vi "Update Progress bar.vi"(10 "Progress Ref":refnum<vi>, 11 "Measurements In":refnum<class "Measurement.lvclass">) -> (3 "Measurements Out":refnum<class "Measurement.lvclass">)   [LabVIEW 2020, in "Measurement.lvclass"]
uses:
  Measurement.lvclass
  Measurement.lvclass/Measurement.ctl
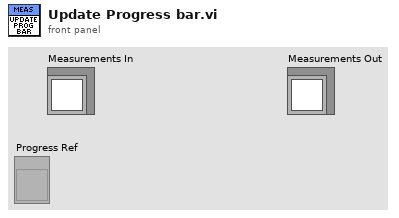
[diagram p1: front panel]
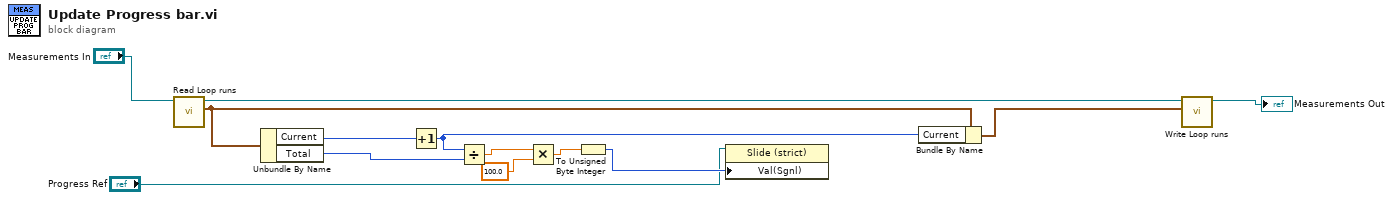
[diagram p0: block diagram]
diagram:
  n1 = call "Read Loop runs.vi"("Measurements in"="Measurements In") -> ("Loop runs"=w3:cluster{"Current":u32, "Total":u32}, "Measurements out"=w4:refnum<class "Measurement.lvclass">)  [unwired: 9 in]
  n2 = Unbundle By Name(w3) -> ("Current"=w6:u32, "Total"=w8:u32)
  n3 = Increment(x=w6) -> (x+1=w7:u32)
  n4 = Divide(x=w7, y=w8) -> (x/y=w9:dbl)
  n5 = Multiply(x=w9, y=100.0) -> (x*y=w11:dbl)
  n6 = To Unsigned Byte Integer(number=w11) -> (unsigned 8bit integer=w13:u8)
  n7 = property class="Slide (strict)"(reference="Progress Ref", "Val(Sgnl)"=w13) -> ()  [unwired: 1 in, 2 out]
  n8 = Bundle By Name(cluster=w3, "Current"=w7) -> (w5:cluster{"Current":u32, "Total":u32})
  n9 = call "Write Loop runs.vi"("Loop runs"=w5, "Measurements in"=w4) -> ("Measurements out"=→"Measurements Out":refnum<class "Measurement.lvclass">)  [unwired: 9 in]
